vi "Pattern Gen TEST.vi"() -> ()   [LabVIEW 2016]
uses:
  Classes/BML_Root/BML_Root.lvclass
  Classes/BML_Root/BML_Root.lvclass/BML_Root.ctl
panel:
  out "error out":errorcluster
  in  "PinMap":path
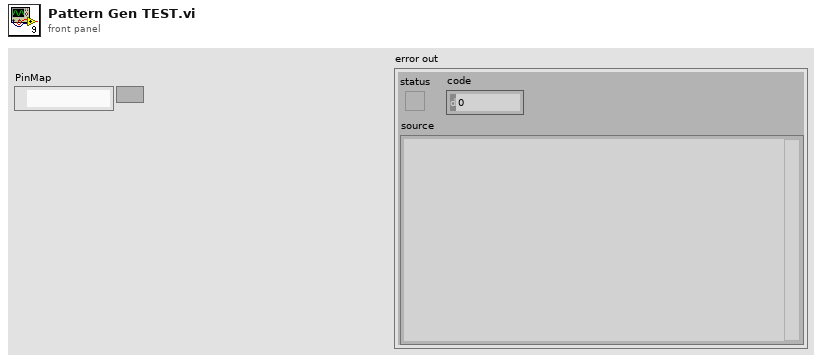
[diagram p1: front panel]
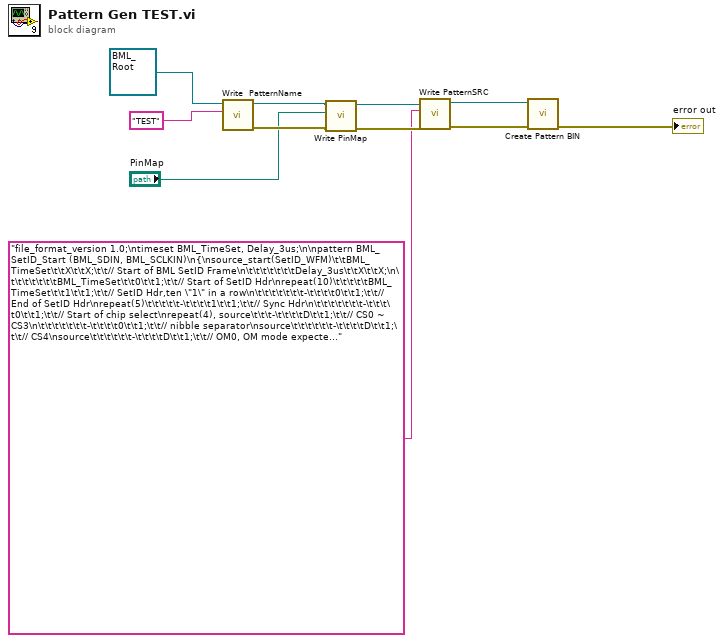
[diagram p0: block diagram]
diagram:
  n1 = call "Write  PatternName.vi"("PatternName"="TEST", "BML_Root in"=refnum<class "BML_Root.lvclass"> refnum ("BML_Root.lvclass")) -> ("error out"=w8:errorcluster, "BML_Root out"=w9:refnum<class "BML_Root.lvclass">)  [unwired: 8 in]
  n2 = call "Write PinMap.vi"("error in (no error)"=w8, "PinMap"="PinMap", "BML_Root in"=w9) -> ("error out"=w5:errorcluster, "BML_Root out"=w6:refnum<class "BML_Root.lvclass">)  [unwired: 7 in]
  n3 = call "Write PatternSRC.vi"("error in (no error)"=w5, "PatternSRC"="file_format_version 1.0;\ntimeset BML_TimeSet, Delay_3us;\n\npattern BML_SetID_Start (BML_SDIN, BML_SCLKIN)\n{\nsource_start(SetID_WFM)\t\tBML_TimeSet\t\tX\t\tX;\t\t// Start of BML SetID Frame\n\t\t\t\t\t\t\tDelay_3us\t\tX\t\tX;\n\t\t\t\t\t\t\tBML_TimeSet\t\t0\t\t1;\t\t// Start of SetID Hdr\nrepeat(10)\t\t\t\t\tBML_TimeSet\t\t1\t\t1;\t\t// SetID Hdr,ten \"1\" in a row\n\t\t\t\t\t\t\t-\t\t\t\t0\t\t1;\t\t// End of SetID Hdr\nrepeat(5)\t\t\t\t\t-\t\t\t\t1\t\t1;\t\t// Sync Hdr\n\t\t\t\t\t\t\t-\t\t\t\t0\t\t1;\t\t// Start of chip select\nrepeat(4), source\t\t\t-\t\t\t\tD\t\t1;\t\t// CS0 ~ CS3\n\t\t\t\t\t\t\t-\t\t\t\t0\t\t1;\t\t// nibble separator\nsource\t\t\t\t\t\t-\t\t\t\tD\t\t1;\t\t// CS4\nsource\t\t\t\t\t\t-\t\t\t\tD\t\t1;\t\t// OM0, OM mode expected to be \"10\"\nsource\t\t\t\t\t\t-\t\t\t\tD\t\t1;\t\t// OM1\nsource\t\t\t\t\t\t-\t\t\t\tD\t\t1;\t\t// R/W?\n\t\t\t\t\t\t\t-\t\t\t\t0\t\t1;\t\t// nibble separator\nrepeat(4), source\t\t\t-\t\t\t\tD\t\t1;\t\t// BL0 ~ BL3\n\t\t\t\t\t\t\t-\t\t\t\t0\t\t1;\t\t// nibble separator\nrepeat(4), source\t\t\t-\t\t\t\tD\t\t1;\t\t// FSN0 ~ FSN3\n\t\t\t\t\t\t\t-\t\t\t\t0\t\t1;\t\t// nibble separator\nhalt\t\t\t\t\t\t-\t\t\t\tX\t\tX;\n}\n", "BML_Root in"=w6) -> ("error out"=w2:errorcluster, "BML_Root out"=w3:refnum<class "BML_Root.lvclass">)  [unwired: 7 in]
  n4 = call "Create Pattern BIN.vi"("error in (no error)"=w2, "BML_Root in"=w3) -> ("error out"=→"error out":errorcluster)  [unwired: 8 in, 1 out]
